vi "lockin.vi"(8 "error in":errorcluster, 10 "NUMERO DE MED.":i32, 11 "milliseconds to wait":u32) -> (0 "error out":errorcluster, 1 "Prom. Voltaje":dbl, 2 "Voltaje":dbl)   [LabVIEW 2018]
uses:
  <vilib>/Instr/_visa.llb/VISA Configure Serial Port (Instr).vi
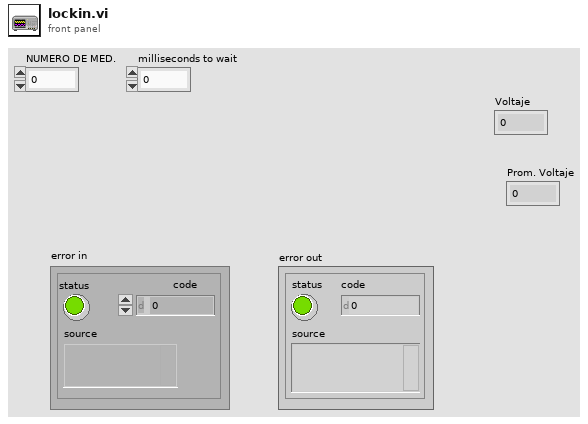
[diagram p1: front panel]
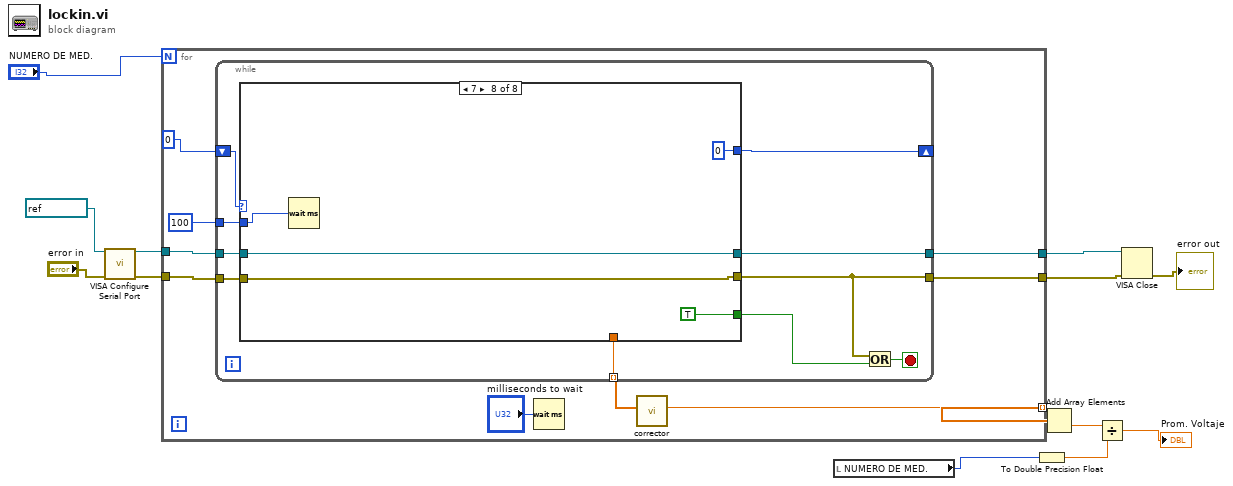
[diagram p0: block diagram]
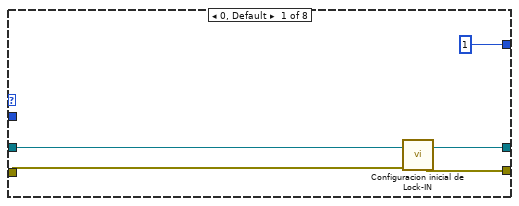
[diagram p2: hidden frame]
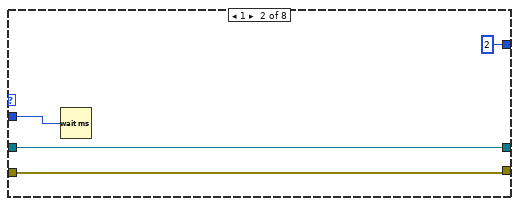
[diagram p3: hidden frame]
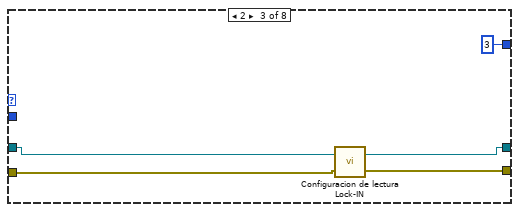
[diagram p4: hidden frame]
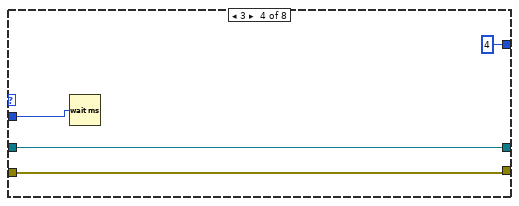
[diagram p5: hidden frame]
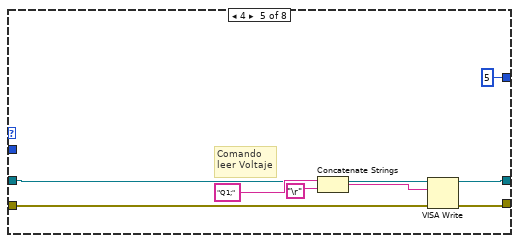
[diagram p6: hidden frame]
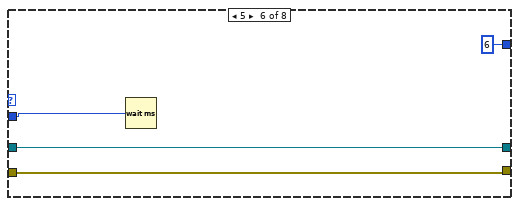
[diagram p7: hidden frame]
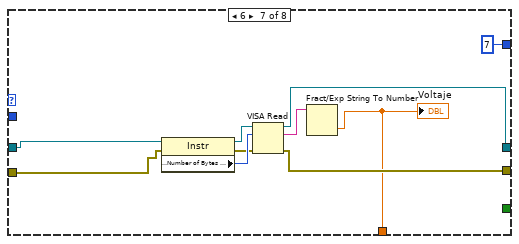
[diagram p8: hidden frame]
diagram:
  n1 = call-poly "VISA Configure Serial Port"("VISA resource name"=refnum<visa-resource-name> "COM4", "error in (no error)"="error in") -> ("VISA resource name out"=w11:refnum<visa-resource-name>, "error out"=w10:errorcluster)  [unwired: 12 in]
  n2 = for {
    N: "NUMERO DE MED." -> [_]
    tunnel: w11 -> [w21]
    tunnel: w10 -> [w20]
    tunnel: [w17] -> w8 mode=indexing
    tunnel: [w15] -> w2
    tunnel: [w14] -> w1
    n3 = while {
      shift-right: [w28] -> _
      shift-left: 0 -> [w32]
      tunnel: w21 -> [w30]
      tunnel: w20 -> [w29]
      tunnel: 100 -> [w27]
      tunnel: [w26] -> w15
      tunnel: [w25] -> w14
      tunnel: [w23] -> w18 mode=indexing
      stop <- w31 stop-if-true
      n4 = case shown="7" w32 {
        tunnel: w30 -> [w37 w39 w46 w49 w54 w61 w68 w76]
        tunnel: w29 -> [w36 w38 w45 w48 w53 w60 w67 w75]
        tunnel: [1 2 3 4 5 6 7 0] -> w28
        tunnel: w27 -> [_ w41 _ w50 _ w62 _ w77]
        tunnel: [w34 w39 w44 w49 w55 w61 w66 w76] -> w26
        tunnel: [w33 w38 w43 w48 w52 w60 w65 w75] -> w25
        tunnel: [_ _ _ _ _ _ _ TRUE] -> w24
        tunnel: [_ _ _ _ _ _ w63 _] -> w23
        frame 0, Default {
          n5 = call "Configuracion inicial de Lock-IN.vi"("error in (no error)"=w36, "VISA resource name"=w37) -> ("error out"=w33:errorcluster, "VISA resource name out"=w34:refnum<visa-resource-name>)
        }
        frame 1 {
          n6 = Wait (ms)(milliseconds to wait=w41) -> ()  [unwired: 1 out]
        }
        frame 2 {
          n7 = call "Configuracion de lectura Lock-IN.vi"("error in (no error)"=w45, "VISA resource name"=w46) -> ("error out"=w43:errorcluster, "VISA resource name out"=w44:refnum<visa-resource-name>)
        }
        frame 3 {
          n8 = Wait (ms)(milliseconds to wait=w50) -> ()  [unwired: 1 out]
        }
        frame 4 {
          # "Comando\nleer Voltaje"
          n9 = Concatenate Strings("Q1;" ("string"), "\r") -> (w56:string)
          n10 = VISA Write(VISA resource name=w54, write buffer=w56, error in (no error)=w53) -> (VISA resource name out=w55:refnum<visa-resource-name>, error out=w52:errorcluster)  [unwired: 1 out]
        }
        frame 5 {
          n11 = Wait (ms)(milliseconds to wait=w62) -> ()  [unwired: 1 out]
        }
        frame 6 {
          n12 = property class="Instr"(reference=w68, error in=w67) -> (reference out=w72:refnum<visa-resource-name>, error out=w70:errorcluster, "Serial Settings:Number of Bytes at Serial Port"=w71:u32)
          n13 = VISA Read(VISA resource name=w72, byte count=w71, error in (no error)=w70) -> (VISA resource name out=w66:refnum<visa-resource-name>, read buffer=w69:string, error out=w65:errorcluster)  [unwired: 1 out]
          n14 = Fract/Exp String To Number(string=w69) -> (number=w63:dbl)  [unwired: 3 in, 1 out]
          "Voltaje" <- w63
        }
        frame 7 {
          n15 = Wait (ms)(milliseconds to wait=w77) -> ()  [unwired: 1 out]
        }
      }
      n16 = Or(x=w25, y=w24) -> (x .or. y?=w31:bool)
    }
    n17 = Wait (ms)(milliseconds to wait="milliseconds to wait") -> ()  [unwired: 1 out]
    n18 = call "corrector.vi"("Array"=w18) -> ("valor salida"=w17:dbl)  [unwired: 10 in]
  }
  n19 = local read "NUMERO DE MED."() -> (w5:i32)
  n20 = To Double Precision Float(number=w5) -> (double precision float=w6:dbl)
  n21 = Add Array Elements(numeric array=w8) -> (sum=w7:dbl)
  n22 = Divide(x=w7, y=w6) -> (x/y=→"Prom. Voltaje":dbl)
  n23 = VISA Close(VISA resource name=w2, error in (no error)=w1) -> (error out=→"error out":errorcluster)
